vi "createDefaultAddDeviceConfig.vi"(8 "error in (no error)":errorcluster, 11 "IDevice in":refnum<class "IDevice.lvclass">) -> (0 "error out":errorcluster, 2 "Config out":refnum<class "IPropertyObject.lvclass">, 3 "IDevice out":refnum<class "IDevice.lvclass">)   [LabVIEW 2022 SP3, in "openDAQ.lvlib" / "IBaseObject.lvlib" / "IPropertyObject.lvlib" / "IComponent.lvlib" / "IFolder.lvlib" / "IDevice.lvlib" / "IDevice.lvclass"]
uses:
  <instrlib>/openDAQ/Public/Classes/IDevice/IDevice.lvclass
  C:/Program Files (x86)/National Instruments/LabVIEW 2022/instr.lib/openDAQ/Public/Classes/IBaseObject/IBaseObject.lvclass
  <instrlib>/openDAQ/Public/Classes/IPropertyObject/IPropertyObject.lvclass
  <instrlib>/openDAQ/Public/Classes/IBaseObject/IBaseObject.lvclass/IBaseObject.ctl
  <instrlib>/openDAQ/Public/Classes/IBaseObject/Accessor/Read reference.vi
  <instrlib>/openDAQ/Public/Classes/IBaseObject/Accessor/Write reference.vi
  <instrlib>/openDAQ/Binaries/Windows/x86/copendaq32.dll
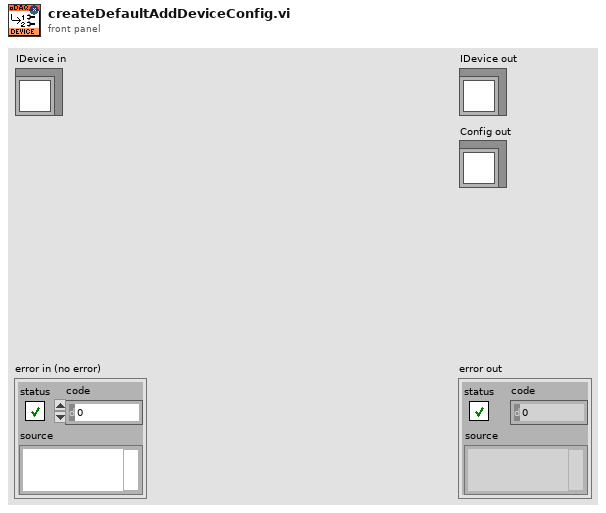
[diagram p1: front panel]
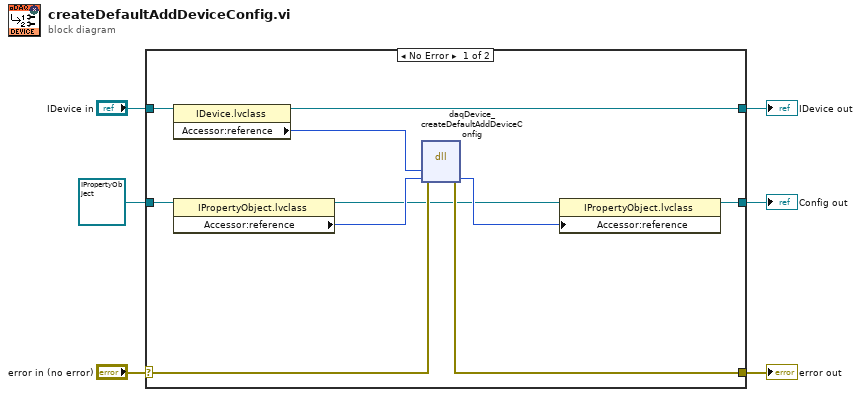
[diagram p0: block diagram]
diagram:
  n1 = case shown="No Error" "error in (no error)" {
    selector: "error in (no error)" -> [w13 w19]
    tunnel: [w12 w19] -> w5
    tunnel: [w11 w18] -> w3
    tunnel: "IDevice in" -> [w15 w18]
    tunnel: refnum<class "IPropertyObject.lvclass"> refnum ("openDAQ.lvlib:IBaseObject.lvlib:IPropertyObject.lvlib:IPropertyObject.lvclass") -> [w10 w17]
    tunnel: [w8 w17] -> w1
    frame No Error {
      n2 = property class="IDevice.lvclass"(reference=w15) -> (reference out=w11:refnum<class "IDevice.lvclass">, "Accessor:reference"=w14:i64)  [unwired: 1 in, 1 out]
      n3 = property class="IPropertyObject.lvclass"(reference=w10) -> (reference out=w7:refnum<class "IPropertyObject.lvclass">, "Accessor:reference"=w9:i64)  [unwired: 1 in, 1 out]
      n4 = dll-call lib="C:/Program Files (x86)/National Instruments/LabVIEW 2022/instr.lib/openDAQ/Binaries/Windows/x86/copendaq*.*" fn="daqDevice_createDefaultAddDeviceConfig"(error in=w13, "device"=w14, "config"=w9) -> (error out=w12:errorcluster, "config"=w16:i64)  [unwired: 4 in, 1 out]
      n5 = property class="IPropertyObject.lvclass"(reference=w7, "Accessor:reference"=w16) -> (reference out=w8:refnum<class "IPropertyObject.lvclass">)  [unwired: 1 in, 1 out]
    }
    frame Error {
    }
  }
  "error out" <- w5
  "IDevice out" <- w3
  "Config out" <- w1
